vi "GraphSetting Get PlotName (Chart).vi"(8 "error in (no error)":errorcluster caption="エラー入力（エラーなし）", 11 "波形チャートref(in)":refnum<vi>) -> (0 "error out":errorcluster caption="エラー出力", 2 "プロット名称[]":string[](array[string]))   [LabVIEW 2014]
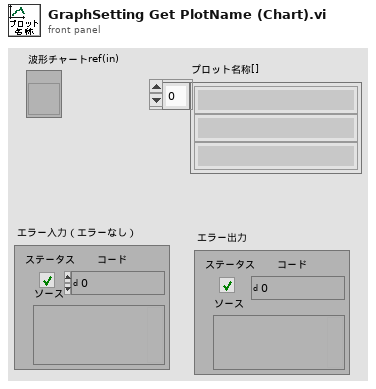
[diagram p1: front panel]
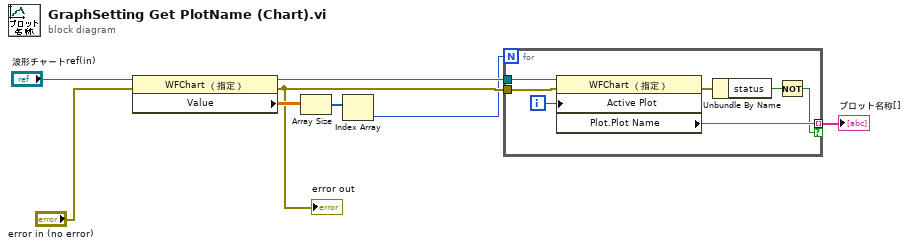
[diagram p0: block diagram]
diagram:
  n1 = property class="WFChart （指定）"(reference="波形チャートref(in)", error in="error in (no error)") -> (reference out=w4:refnum<vi>, error out=w2:errorcluster, "Value"=w6:dbl[][])
  "error out" <- w2
  n2 = Array Size(array=w6) -> (size(s)=w5:i32[])
  n3 = Index Array(array=w5) -> (element=w1:i32)  [unwired: 1 in]
  n4 = for {
    N: w1 -> [_]
    tunnel: w4 -> [w15]
    tunnel: [w13] -> w8 mode=indexing if=w10
    tunnel: w2 -> [w9]
    i -> [w14]
    n5 = property class="WFChart （指定）"(reference=w15, error in=w9, "Active Plot"=w14) -> (error out=w12:errorcluster, "Plot.Plot Name"=w13:string)  [unwired: 1 out]
    n6 = Unbundle By Name(w12) -> ("status"=w11:bool)
    n7 = Not(x=w11) -> (.not. x?=w10:bool)
  }
  "プロット名称[]" <- w8
